vi "ex_Make Hidden Tag.vi"(1 "Tag Name":string) -> (0 "Hidden Tag Name":string)   [LabVIEW 2017]
doc: "Takes an input string and adds an underscore character to the beginning of it."
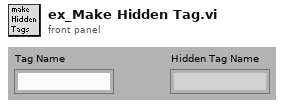
[diagram p1: front panel]
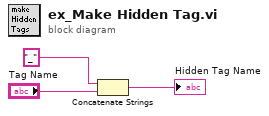
[diagram p0: block diagram]
diagram:
  n1 = Concatenate Strings("_" ("Substring"), "Tag Name") -> (→"Hidden Tag Name":string)
